vi "PH_Sequencer.evt call Clear Z6 Beamline.vi"(0 "i ref in":refnum<vi>, 2 "Instance":string="N/A", 5 "error in (no error)":errorcluster) -> (14 "i ref out":refnum<vi>, 19 "error out":errorcluster)   [LabVIEW 2014, in "PH_Sequencer.lvlib"]
doc: "This VI calls the case \"ClearZ6Beamline\" by a simple call."
uses:
  PH_Sequencer.lvlib
  CSCore/BaseProcess/BaseProcess.lvlib
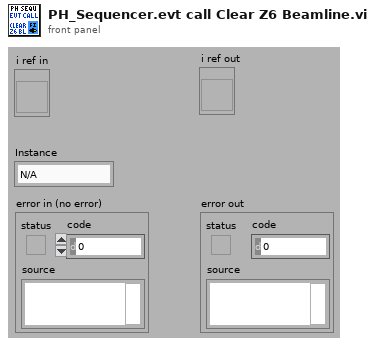
[diagram p1: front panel]
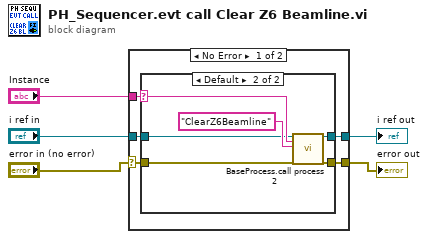
[diagram p0: block diagram]
diagram:
  n1 = case shown="No Error" "error in (no error)" {
    selector: "error in (no error)" -> [w8 w20]
    tunnel: [w10 w19] -> w2
    tunnel: [w9 w20] -> w1
    tunnel: "i ref in" -> [w7 w19]
    tunnel: "Instance" -> [w6 _]
    frame No Error {
      n2 = case shown="Default" w6 {
        selector: w6 -> [_ w14]
        tunnel: [w11 w18] -> w10
        tunnel: [w12 w17] -> w9
        tunnel: w8 -> [w12 w16]
        tunnel: w7 -> [w11 w13]
        frame "N/A" {
        }
        frame Default {
          n3 = call "BaseProcess.call process 2.vi"("i ref in"=w13, "Object"=w14, "Selector"="ClearZ6Beamline", "error in (no error)"=w16) -> ("i ref out"=w18:refnum<vi>, "error out"=w17:errorcluster)  [unwired: 14 in]
        }
      }
    }
    frame Error {
    }
  }
  "error out" <- w1
  "i ref out" <- w2
